vi "counter_meas.vi"(7 "error in (no error)":errorcluster, 9 "Kalibracni bod":T1, 10 "VISA Refnum in":refnum<visa-resource-name>) -> (0 "error out":errorcluster, 1 "number":dbl, 2 "Raw data":string, 3 "VISA Refnum out":refnum<visa-resource-name>)   [LabVIEW 2022 SP3]
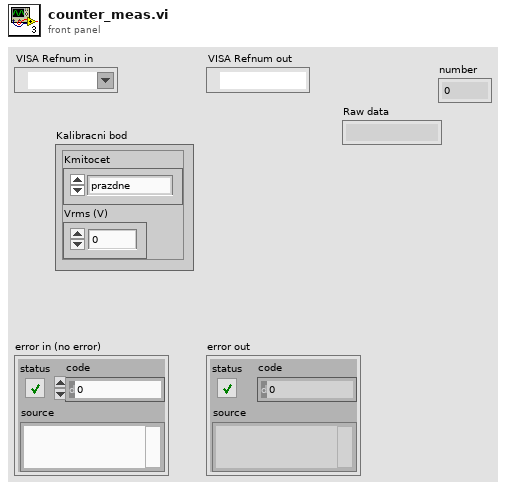
[diagram p1: front panel]
types:
  T1 = cluster{"Kmitocet":enum16{"prazdne", "50 Hz", "1 kHz", "5 kHz", "10 kHz", "20 kHz", "50 kHz", "100 kHz"}, "Vrms (V)":dbl}
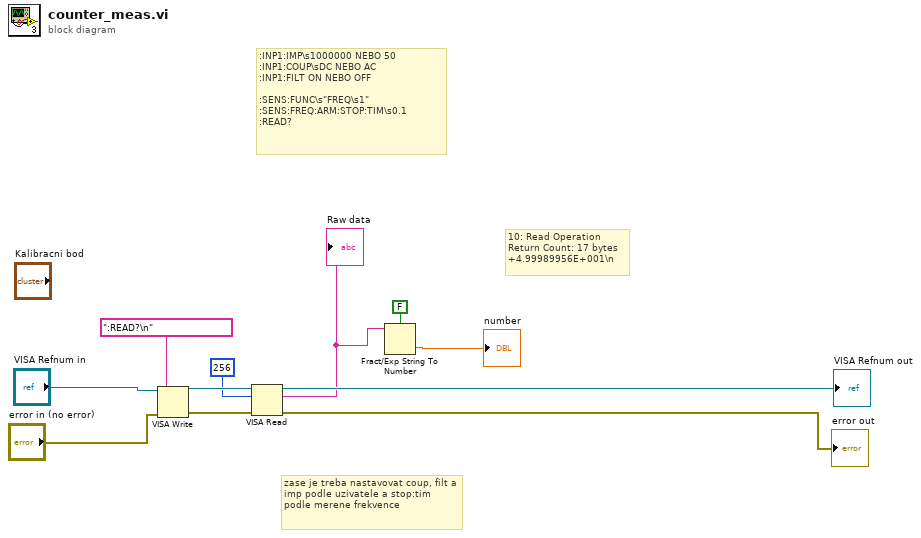
[diagram p0: block diagram]
diagram:
  # "10: Read Operation\nReturn Count: 17 bytes\n+4.99989956E+001\\n"
  # ":INP1:IMP\\s1000000 NEBO 50\n:INP1:COUP\\sDC NEBO AC\n:INP1:FILT ON NEBO OFF\n\n:SENS:FUNC\\s\"FREQ\\s1\"\n:SENS:FREQ:ARM:STOP:TIM\\s0.1\n:READ?"
  # "zase je treba nastavovat coup, filt a imp podle uzivatele a stop:tim podle merene frekvence"
  n1 = VISA Write(VISA resource name="VISA Refnum in", write buffer=":READ?\n", error in (no error)="error in (no error)") -> (VISA resource name out=w8:refnum<visa-resource-name>, error out=w5:errorcluster)  [unwired: 1 out]
  n2 = VISA Read(VISA resource name=w8, byte count=u32 256, error in (no error)=w5) -> (VISA resource name out=→"VISA Refnum out":refnum<visa-resource-name>, read buffer=w1:string, error out=→"error out":errorcluster)  [unwired: 1 out]
  "Raw data" <- w1
  n3 = Fract/Exp String To Number(use system decimal point (T)=FALSE, string=w1) -> (number=→"number":dbl)  [unwired: 2 in, 1 out]
